vi "Test Report Contain Passing TestCase Name.vi"(8 "error in (no error)":errorcluster, 11 "XML Report Test in":refnum<class "XML Report Test.lvclass">) -> (0 "error out":errorcluster, 3 "XML Report Test out":refnum<class "XML Report Test.lvclass">)   [LabVIEW 2020, in "XML Report Test.lvclass"]
uses:
  XML Report Test.lvclass
  source/Plugins/XML Report/XML Report.lvclass
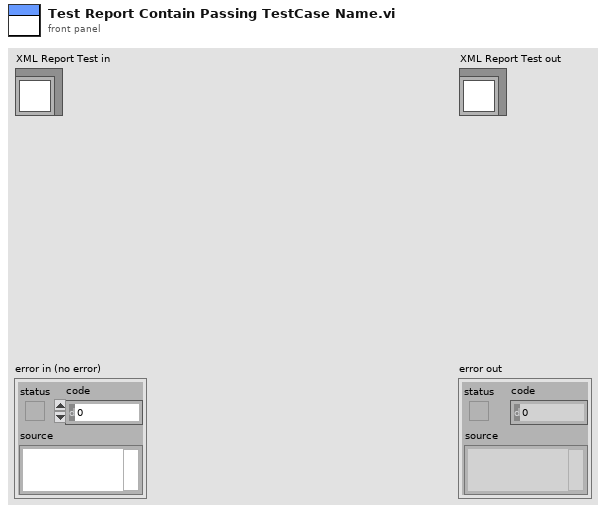
[diagram p1: front panel]
types:
  T1 = typedef "Result.lvlib/Result.ctl" = cluster{"Name":string, "Message":string, "Description":string, "Status":T2, "Result Type":T3, "Execution Time":dbl}
  T2 = typedef "Result.lvlib/Status.ctl" = enum16{"", "Passed", "Failed", "Error", "Skipped", "Setup Error", "Broken", "Teardown Error"}
  T3 = typedef "Result.lvlib/Type.ctl" = enum16{"Method", "Case", "Suite", "Pass", "Fail", "Skip", "Pass if", "Fail if", "Pass if Error", "Fail if Error", "Pass if Equal", "Fail if Equal"}
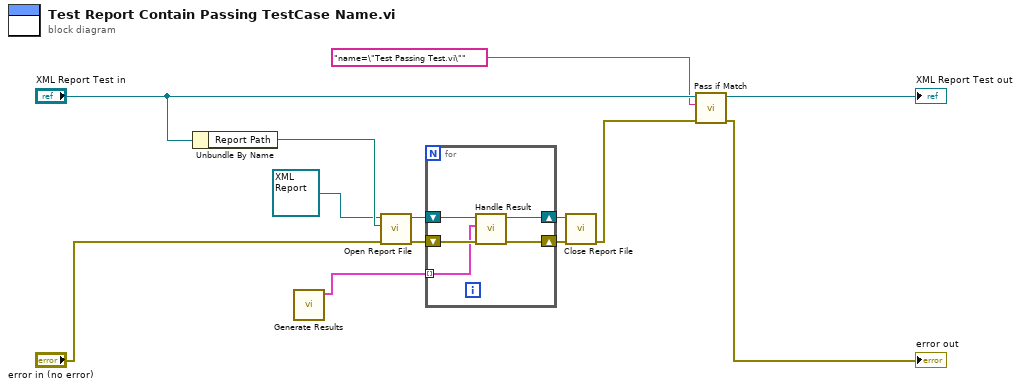
[diagram p0: block diagram]
diagram:
  n1 = Unbundle By Name("XML Report Test in") -> ("Report Path"=w7:path)
  n2 = call "Generate Results.vi"() -> ("Data"=w1:T1[])  [unwired: 10 in, 1 out]
  n3 = call-dynamic "Open Report File.vi"("error in (no error)"="error in (no error)", "Report Path"=w7, "XML Report In"=refnum<class "XML Report.lvclass"> refnum) -> ("error out"=w13:errorcluster, "XML Report Out"=w3:refnum<class "XML Report.lvclass">)  [unwired: 7 in]
  n4 = for {
    shift-right: [w17] -> w4
    shift-left: w13 -> [w18]
    shift-right: [w15] -> w2
    shift-left: w3 -> [w16]
    tunnel: w1 -> [w14] mode=indexing
    n5 = call-dynamic "Handle Result.vi"("error in (no error)"=w18, "Result"=w14, "XML Report In"=w16) -> ("error out"=w17:errorcluster, "XML Report Out"=w15:refnum<class "XML Report.lvclass">)  [unwired: 7 in]
  }
  n6 = call-dynamic "Close Report File.vi"("error in (no error)"=w4, "XML Report In"=w2) -> ("error out"=w9:errorcluster)  [unwired: 9 in]
  n7 = call "Pass if Match.vi"("error in (no error)"=w9, "regular expression"="name=\"Test Passing Test.vi\"", "XML Report Test in"="XML Report Test in") -> ("error out"=→"error out":errorcluster, "XML Report Test out"=→"XML Report Test out":refnum<class "XML Report Test.lvclass">)  [unwired: 6 in, 1 out]
